vi "Name for Folder.vi"(8 "error in (no error)":errorcluster, 10 "Folder":path, 11 "PackageAbstract in":refnum<class "PackageAbstract.lvclass">) -> (0 "error out":errorcluster, 1 "Name":string, 2 "Folder dup":path, 3 "PackageAbstract out":refnum<class "PackageAbstract.lvclass">)   [LabVIEW 2020, in "GPack.lvlib" / "PackageAbstract.lvclass"]
uses:
  PackageAbstract.lvclass
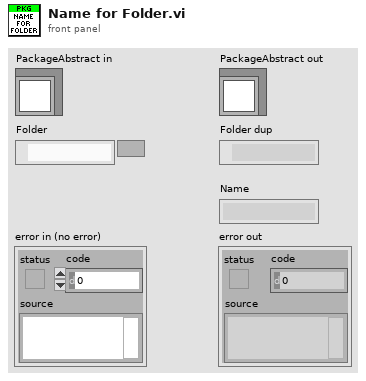
[diagram p1: front panel]
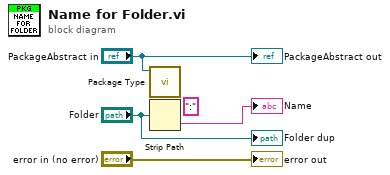
[diagram p0: block diagram]
diagram:
  (unwired) ":" ("string")
  n1 = call-dynamic "Package Type.vi"("PackageInfo in"="PackageAbstract in") -> ()  [unwired: 9 in, 2 out]
  n2 = Strip Path(path="Folder") -> (name=→"Name":string)  [unwired: 1 out]
  "error out" <- "error in (no error)"
  "PackageAbstract out" <- "PackageAbstract in"
  "Folder dup" <- "Folder"
